vi "OpenProj.vi"(11 "Command line arguments for the VI":string[](array[string])) -> (2 "Output or error information to include in the CLI for LabVIEW console or log file.":string, 3 "CLI for LabVIEW exit code that the VI returns":i32)   [LabVIEW 2020]
doc: "This VI opens the project window given its absolute path. It is meant to be used with LabVIEWCLI."
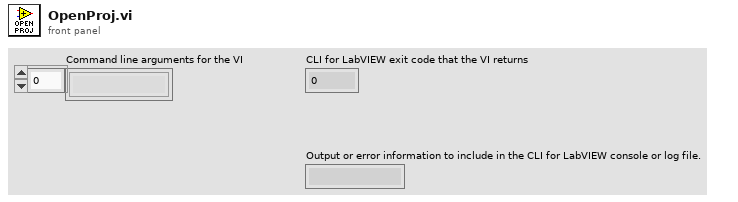
[diagram p1: front panel]
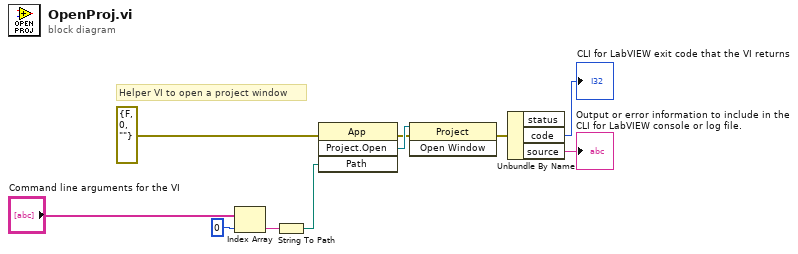
[diagram p0: block diagram]
diagram:
  # "Helper VI to open a project window"
  n1 = Index Array(array="Command line arguments for the VI", index=0) -> (element=w7:string)
  n2 = String To Path(string=w7) -> (path=w6:path)
  n3 = invoke on="Invoke Node" class="App" method="Project.Open"(error in=errorcluster {"status"=FALSE, "code"=0, "source"=""} ("error constant"), "Path"=w6) -> (error out=w4:errorcluster, "Project:Open"=w10:refnum<vi>)  [unwired: 2 in, 2 out]
  n4 = invoke on="Invoke Node" class="Project" method="Open Window"(reference=w10, error in=w4) -> (error out=w3:errorcluster)  [unwired: 1 in, 2 out]
  n5 = Unbundle By Name(w3) -> ("code"=→"CLI for LabVIEW exit code that the VI returns":i32, "source"=→"Output or error information to include in the CLI for LabVIEW console or log file.":string)  [unwired: 1 out]
